vi "list.count.vi"(8 "error in":errorcluster, 11 "List in":refnum<class "List.lvclass">) -> (0 "error out":errorcluster, 2 "count":u32, 3 "List out":refnum<class "List.lvclass">)   [LabVIEW 2020, in "List.lvclass"]
uses:
  List.lvclass
  List.lvclass/List.ctl
  client.lvlib
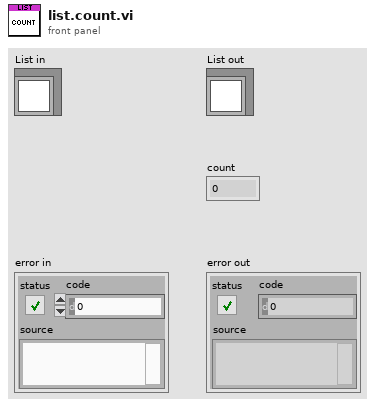
[diagram p1: front panel]
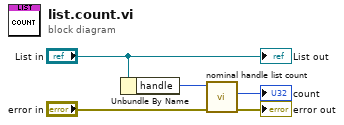
[diagram p0: block diagram]
diagram:
  n1 = Unbundle By Name("List in") -> ("handle"=w1:i32)
  n2 = call "nominal handle list count.vi"("error in (no error)"="error in", "list"=w1) -> ("error out"=→"error out":errorcluster, "out_count out"=→"count":u32)  [unwired: 7 in, 1 out]
  "List out" <- "List in"
